vi "Update Car Instance.vi"(7 "Car Name":string, 8 "error in (no error)":errorcluster, 10 "Car":refnum<class "Car.lvclass">, 11 "CarPool in":refnum<class "CarPool.lvclass">) -> (0 "error out":errorcluster, 3 "CarPool out":refnum<class "CarPool.lvclass">)   [LabVIEW 2017, in "CarPool.lvclass"]
uses:
  CarPool.lvclass
  Car/Car.lvclass
  CarPool.lvclass/CarPool.ctl
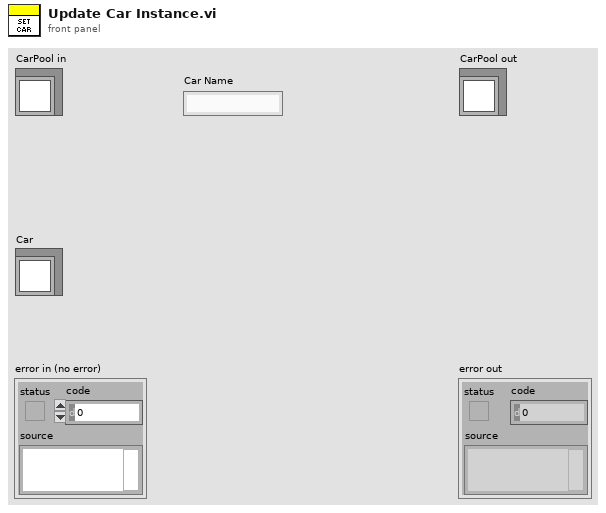
[diagram p1: front panel]
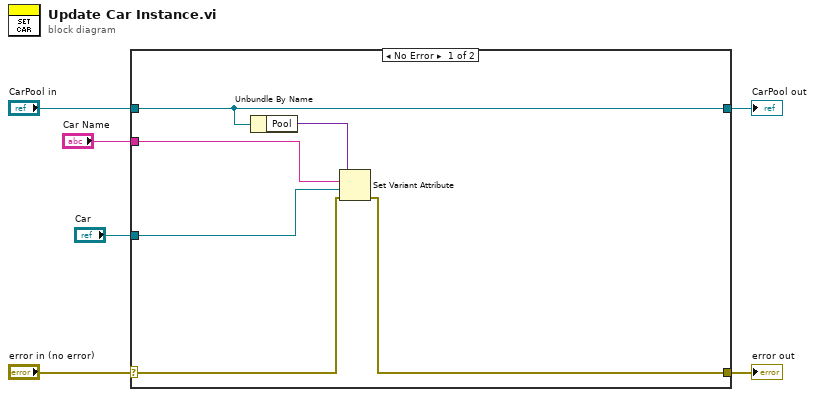
[diagram p0: block diagram]
diagram:
  n1 = case shown="No Error" "error in (no error)" {
    selector: "error in (no error)" -> [w9 w14]
    tunnel: [w8 w14] -> w5
    tunnel: [w11 w13] -> w3
    tunnel: "CarPool in" -> [w11 w13]
    tunnel: "Car Name" -> [w12 _]
    tunnel: "Car" -> [w7 _]
    frame No Error {
      n2 = Unbundle By Name(w11) -> ("Pool"=w10:variant)
      n3 = Set Variant Attribute(Variant=w10, name=w12, value=w7, error in=w9) -> (error out=w8:errorcluster)  [unwired: 2 out]
    }
    frame Error {
    }
  }
  "error out" <- w5
  "CarPool out" <- w3
